vi "Logging Deduplicate Unsaved.vi"(1 "Input":cluster{"Variable":T1, "refnum":refnum<file>}[](array[cluster])) -> (0 "Output":cluster{"Variable":T1, "refnum":refnum<file>}[](array[cluster]))   [LabVIEW 2012, in "femtoRoboLib.lvlib"]
uses:
  femtoRoboLib.lvlib
  Controls/Log Entry - Converted.ctl
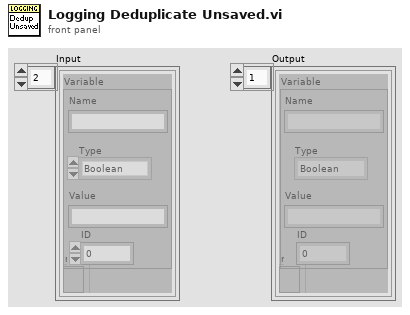
[diagram p1: front panel]
types:
  T1 = typedef "femtoRoboLib.lvlib/Log Entry - Converted.ctl" = cluster{"Name":string, "Type":enum16{"Boolean", "Numeric", "String", "Boolean Array", "Numeric Array", "String Array"}, "Value":string, "ID":u32}
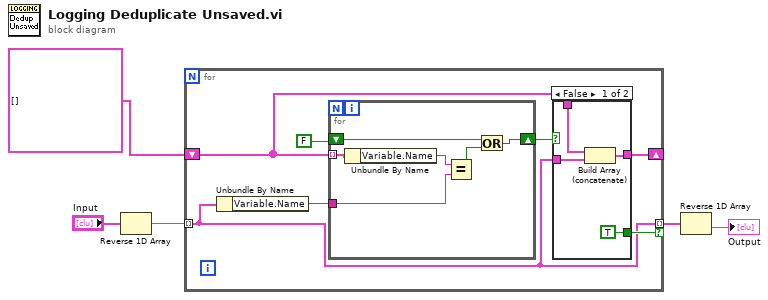
[diagram p0: block diagram]
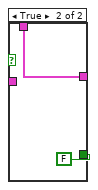
[diagram p2: hidden frame]
diagram:
  n1 = Reverse 1D Array(array="Input") -> (reversed array=w3:cluster{"Variable":T1, "refnum":refnum<file>}[])
  n2 = for {
    tunnel: w3 -> [w6] mode=indexing
    shift-right: [w8] -> _
    shift-left: cluster{"Variable":T1, "refnum":refnum<file>}[] [] ("reversed array") -> [w9]
    tunnel: [w6] -> w1 mode=indexing if=w7
    n3 = Unbundle By Name(w6) -> ("Variable.Name"=w11:string)
    n4 = for {
      shift-right: [w20] -> w10
      shift-left: FALSE -> [w24]
      tunnel: w9 -> [w19] mode=indexing
      tunnel: w11 -> [w21]
      n5 = Unbundle By Name(w19) -> ("Variable.Name"=w22:string)
      n6 = Equal?(x=w22, y=w21) -> (x = y?=w23:bool)
      n7 = Or(x=w24, y=w23) -> (x .or. y?=w20:bool)
    }
    n8 = case shown="False" w10 {
      tunnel: w9 -> [w16 w18]
      tunnel: [w15 w18] -> w8
      tunnel: [TRUE FALSE] -> w7
      tunnel: w6 -> [w13 _]
      frame False {
        n9 = Build Array (concatenate)(w16, w13) -> (w15:cluster{"Variable":T1, "refnum":refnum<file>}[])
      }
      frame True {
      }
    }
  }
  n10 = Reverse 1D Array(array=w1) -> (reversed array=→"Output":cluster{"Variable":T1, "refnum":refnum<file>}[])
